vi "piezoWriteWriteFuncGenNew.vi"() -> ()   [LabVIEW 2017]
doc: "Starts the piezo with a triangle or sine wave in continuous mode."
uses:
  <vilib>/DAQmx/write.llb/DAQmx Write (Analog 1D DBL 1Chan NSamp).vi
  globalDevices.vi
  globalUtilities.vi
  <vilib>/DAQmx/miscellaneous.llb/DAQmx Fill In Error Info.vi
panel:
  out "Waveform Graph 4":dbl[](graph)
  out "success":bool
  out "Waveform Graph 3":dbl[](graph)
  out "nT":i32
  out "dt":dbl
  out "omega":dbl
  out "amplitude":dbl
  out "offset":dbl
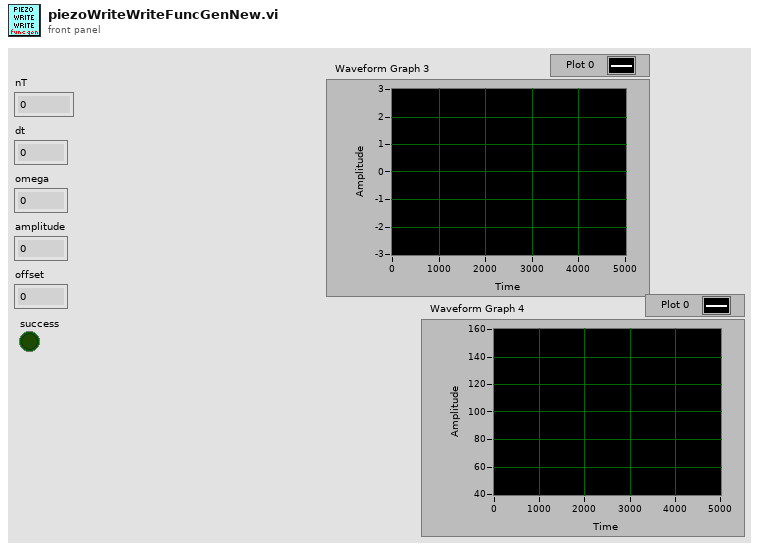
[diagram p1: front panel]
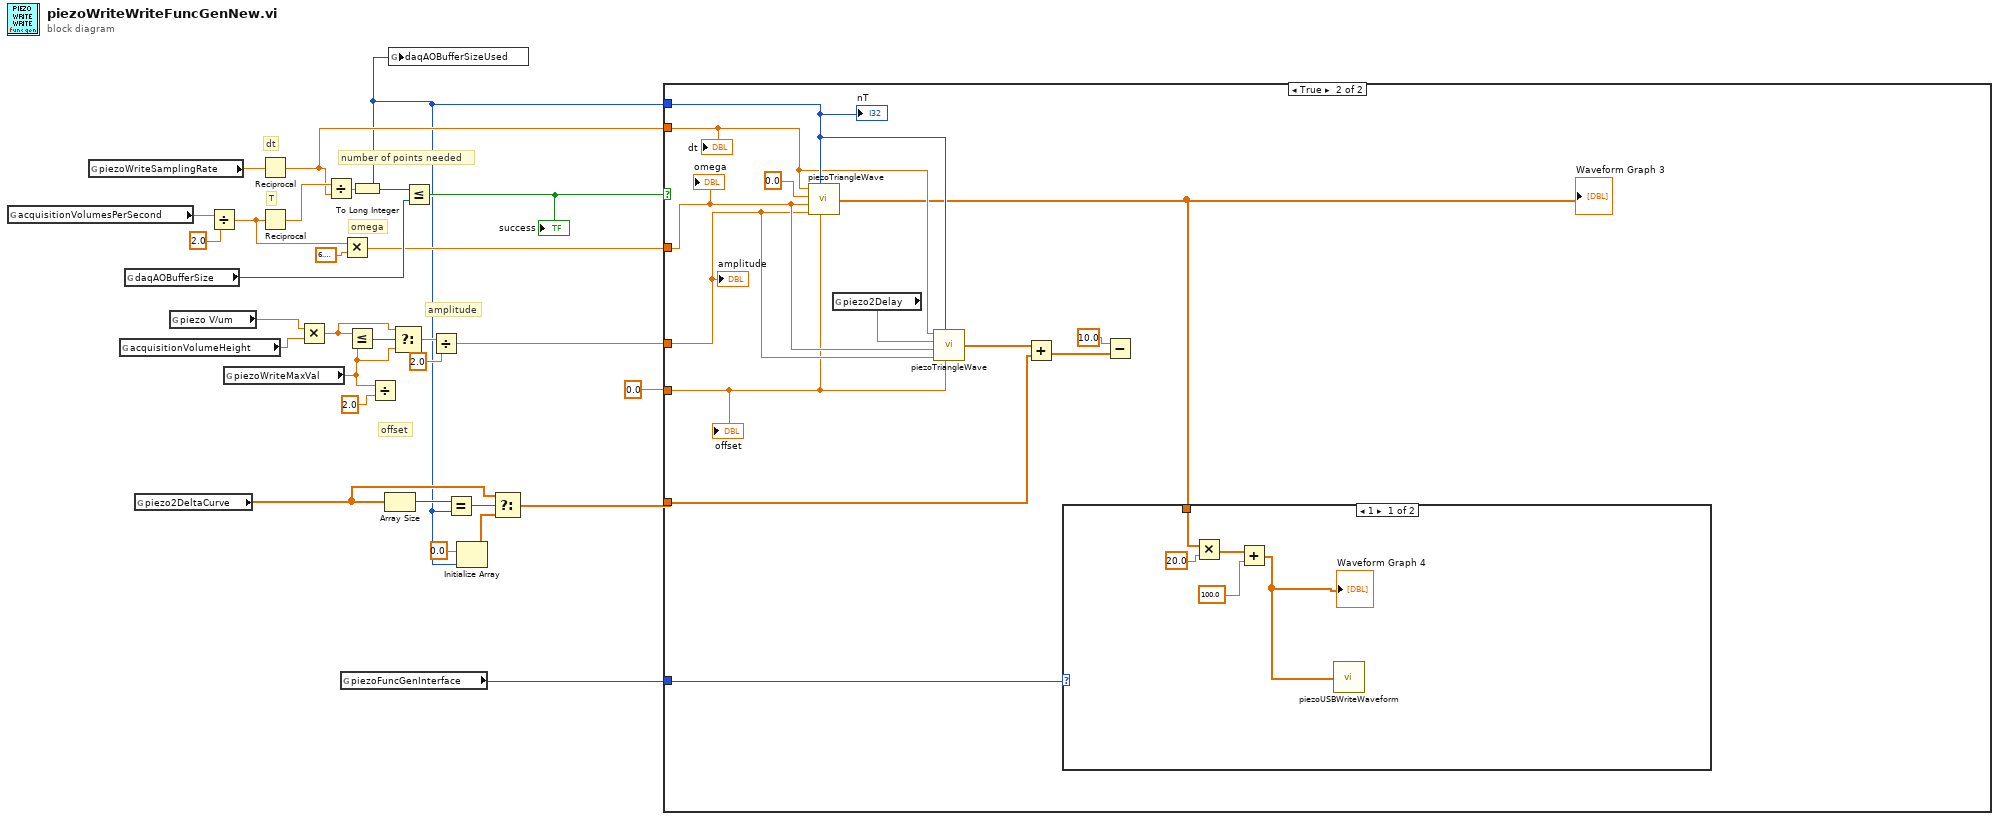
[diagram p0: block diagram]
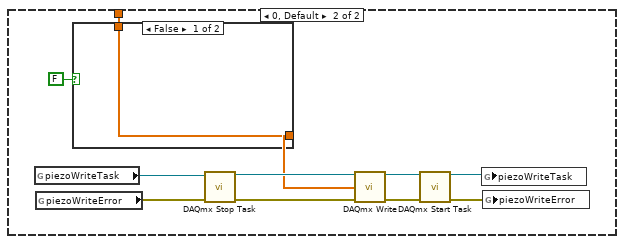
[diagram p3: hidden frame]
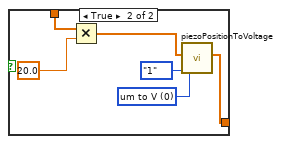
[diagram p4: hidden frame]
diagram:
  # "omega"
  # "amplitude"
  # "offset"
  # "number of points needed"
  # "T"
  # "dt"
  n1 = global read "globalUtilities.vi" "acquisitionVolumesPerSecond"() -> (w28:dbl)
  n2 = global read "globalDevices.vi" "piezoWriteSamplingRate"() -> (w29:dbl)
  n3 = global read "globalUtilities.vi" "acquisitionVolumeHeight"() -> (w22:dbl)
  n4 = global read "globalDevices.vi" "daqAOBufferSize"() -> (w25:i32)
  n5 = global read "globalDevices.vi" "piezo2DeltaCurve"() -> (w8:dbl[])
  n6 = global read "globalDevices.vi" "piezo V/um"() -> (w23:dbl)
  n7 = Divide(x=w28, y=2.0) -> (x/y=w13:dbl)
  n8 = global read "globalDevices.vi" "piezoWriteMaxVal"() -> (w19:dbl)
  n9 = Reciprocal(x=w29) -> (1/x=w11:dbl)
  n10 = Reciprocal(x=w13) -> (1/x=w26:dbl)
  n11 = Multiply(x=w23, y=w22) -> (x*y=w20:dbl)
  n12 = Divide(x=w26, y=w11) -> (x/y=w4:dbl)
  n13 = global read "globalDevices.vi" "piezoFuncGenInterface"() -> (w1:u16)
  n14 = Multiply(x=w13, y=6.283185307179586) -> (x*y=w12:dbl)
  n15 = Less Or Equal?(x=w20, y=w19) -> (x <= y?=w21:bool)
  n16 = To Long Integer(number=w4) -> (32bit integer=w3:i32)
  n17 = Divide(x=w19, y=2.0) -> ()  [unwired: 1 out]
  n18 = Array Size(array=w8) -> (size(s)=w10:i32)
  n19 = global write "globalDevices.vi" "daqAOBufferSizeUsed"(w3) -> ()
  n20 = Select(t=w20, s=w21, f=w19) -> (s? t:f=w17:dbl)
  n21 = Less Or Equal?(x=w3, y=w25) -> (x <= y?=w24:bool)
  "success" <- w24
  n22 = Divide(x=w17, y=2.0) -> (x/y=w15:dbl)
  n23 = Equal?(x=w10, y=w3) -> (x = y?=w9:bool)
  n24 = Initialize Array(0.0 ("element"), w3) -> (w6:dbl[])
  n25 = Select(t=w8, s=w9, f=w6) -> (s? t:f=w5:dbl[])
  n26 = case shown="True" w24 {
    tunnel: w15 -> [_ w37]
    tunnel: 0.0 -> [_ w36]
    tunnel: w12 -> [_ w38]
    tunnel: w3 -> [_ w41]
    tunnel: w11 -> [_ w40]
    tunnel: w5 -> [_ w34]
    tunnel: w1 -> [_ w30]
    frame False {
    }
    frame True {
      n27 = call "piezoTriangleWave.vi"("offset"=w36, "nT"=w41, "amplitude"=w37, "omega"=w38, "t0"=0.0, "dt"=w40) -> ("x+y"=w31:dbl[])
      "Waveform Graph 3" <- w31
      n28 = global read "globalDevices.vi" "piezo2Delay"() -> (w39:dbl)
      n29 = call "piezoTriangleWave.vi"("offset"=w36, "nT"=w41, "amplitude"=w37, "omega"=w38, "t0"=w39, "dt"=w40) -> ("x+y"=w35:dbl[])
      n30 = Add(x=w35, y=w34) -> (x+y=w33:dbl[])
      n31 = case shown="1" w30 {
        tunnel: w31 -> [w47 w50]
        frame 1 {
          n32 = Multiply(x=w47, y=20.0) -> (x*y=w45:dbl[])
          n33 = Add(x=w45, y=100.0) -> (x+y=w43:dbl[])
          "Waveform Graph 4" <- w43
          n34 = call "piezoUSBWriteWaveform.vi"("positions (um)"=w43) -> ()  [unwired: 1 in]
        }
        frame 0, Default {
          n35 = global read "globalDevices.vi" "piezoWriteTask"() -> (w52:refnum<k21>)
          n36 = global read "globalDevices.vi" "piezoWriteError"() -> (w51:errorcluster)
          n37 = case shown="False" FALSE {
            tunnel: w50 -> [w59 w65]
            tunnel: [w59 w60] -> w49
            frame False {
            }
            frame True {
              w61 = u16 0 items=["um to V", "V to um"] ("mode")
              n38 = Multiply(x=w65, y=20.0) -> (x*y=w63:dbl[])
              n39 = call "piezoPositionToVoltage.vi"("piezo"=enum16{"1", "2"}."1", "mode"=w61, "in (array)"=w63) -> ("out (array)"=w60:dbl[])  [unwired: 3 in, 1 out]
            }
          }
          n40 = call <vilib>:"DAQmx Stop Task.vi"("task/channels in"=w52, "error in"=w51) -> ("task out"=w53:refnum<k21>, "error out"=w54:errorcluster)  [unwired: 12 in]
          n41 = call-poly <vilib>:"DAQmx Write.vi"("task/channels in"=w53, "data"=w49, "error in"=w54) -> ("task out"=w57:refnum<k21>, "error out"=w58:errorcluster)  [unwired: 10 in, 1 out]
          n42 = call <vilib>:"DAQmx Start Task.vi"("task/channels in"=w57, "error in"=w58) -> ("task out"=w55:refnum<k21>, "error out"=w56:errorcluster)  [unwired: 12 in]
          n43 = global write "globalDevices.vi" "piezoWriteTask"(w55) -> ()
          n44 = global write "globalDevices.vi" "piezoWriteError"(w56) -> ()
        }
      }
      n45 = Subtract(x=10.0, y=w33) -> ()  [unwired: 1 out]
      "nT" <- w41
      "dt" <- w40
      "omega" <- w38
      "amplitude" <- w37
      "offset" <- w36
    }
  }
